vi "DHE_GetAlgorsFile.vi"() -> (7 "DHE_AlgorsFile":path)   [LabVIEW 2016]
uses:
  private/vis/DHE_GBLDriverVariables.vi
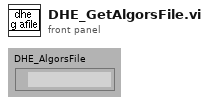
[diagram p1: front panel]
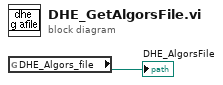
[diagram p0: block diagram]
diagram:
  n1 = global read "DHE_GBLDriverVariables.vi" "DHE_Algors_file"() -> (→"DHE_AlgorsFile":path)
